vi "S7_Optimize_DB_Read_Array.vi"(2 "S7 Read Array Input":T3[](array[typedef]) {"Address Areas" items=["I/O (P)"=128, "Input (I)"=129, "Output (Q)"=130, "Bit Memory (M)"=131, "Data (DB)"=132, "Instance Data (DI)"=133, "Local Data (L)"=134, "Predecessor Local Data (VL)"=135]; "Read / Write" items=["Read"=4, "Write"=5]; "Bit Number / Byte Length" max=7 step=1}, 3 "Max Size":u8=222) -> (0 "Optimized Data Index":T1[](array[typedef]) {"Bit Number" max=7 step=1}, 1 "Optimized S7 Read Array Output":T3[](array[typedef]) {"Address Areas" items=["I/O (P)"=128, "Input (I)"=129, "Output (Q)"=130, "Bit Memory (M)"=131, "Data (DB)"=132, "Instance Data (DI)"=133, "Local Data (L)"=134, "Predecessor Local Data (VL)"=135]; "Read / Write" items=["Read"=4, "Write"=5]; "Bit Number / Byte Length" max=7 step=1})   [LabVIEW 2014, in "S7 TCP.lvlib"]
uses:
  S7 TCP.lvlib
  Data Type.ctl
  S7 Read Write Cluster.ctl
  Optimized Data Index.ctl
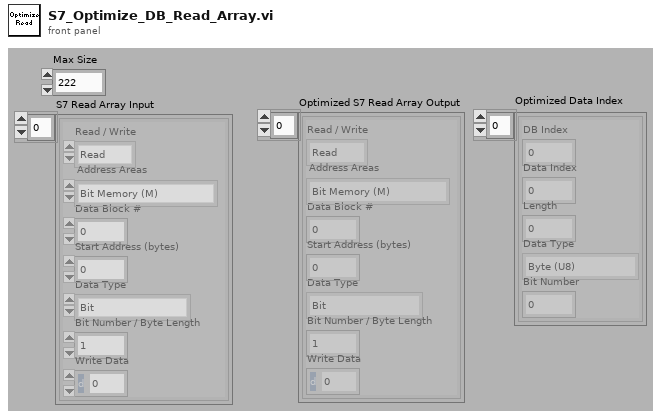
[diagram p1: front panel]
types:
  T1 = typedef "S7 TCP.lvlib/Optimized Data Index.ctl" = cluster{"DB Index":i32, "Data Index":i32, "Length":i32, "Data Type":T2, "Bit Number":u8}
  T2 = typedef "S7 TCP.lvlib/Data Type.ctl" = enum16{"Bit", "Byte (U8)", "Signed Byte (I8)", "Word (U16)", "Signed Word (I16)", "Long (U32)", "Signed Long (I32)", "Real (SGL)", "Defined Byte Length"}
  T3 = typedef "S7 TCP.lvlib/S7 Read Write Cluster.ctl" = cluster{"Read / Write":u8, "Address Areas":u8, "Data Block #":u16, "Start Address (bytes)":u32, "Data Type":T2, "Bit Number / Byte Length":u8, "Write Data":dbl}
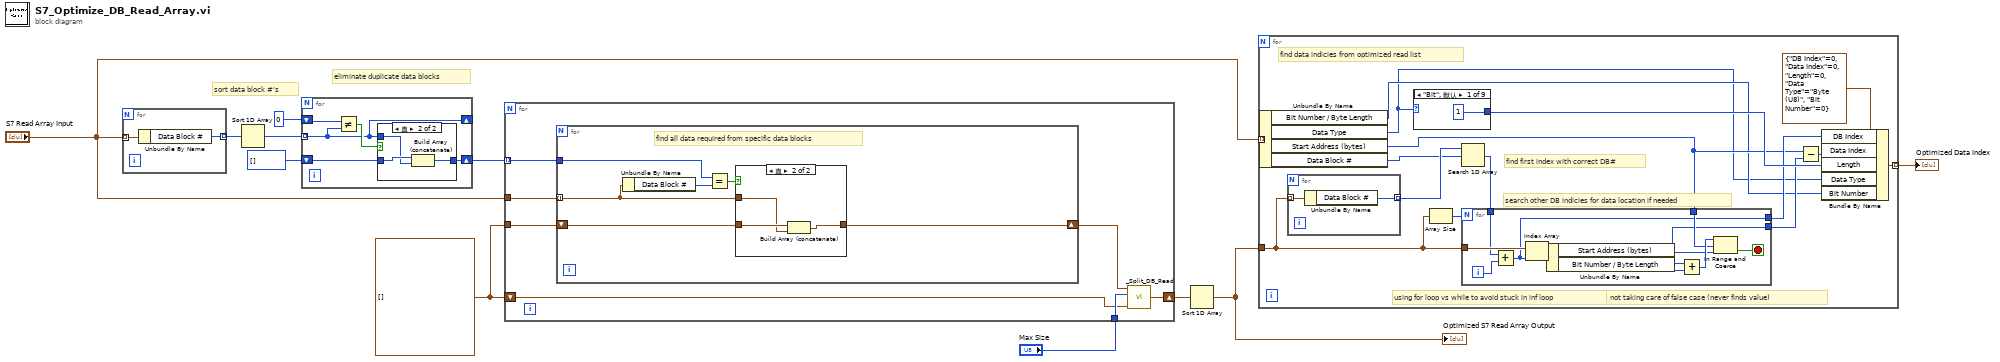
[diagram p0: block diagram]
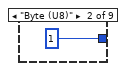
[diagram p2: hidden frame]
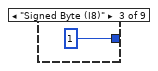
[diagram p3: hidden frame]
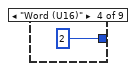
[diagram p4: hidden frame]
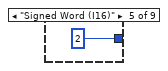
[diagram p5: hidden frame]
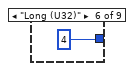
[diagram p6: hidden frame]
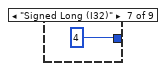
[diagram p7: hidden frame]
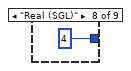
[diagram p8: hidden frame]
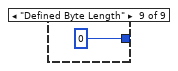
[diagram p9: hidden frame]
diagram:
  w2 = T3[] [] ("Optimized S7 Read Array Output 2")
  # "eliminate duplicate data blocks"
  # "sort data block #'s"
  n1 = for {
    tunnel: "S7 Read Array Input" -> [w13] mode=indexing
    tunnel: [w12] -> w11 mode=indexing
    n2 = Unbundle By Name(w13) -> ("Data Block #"=w12:u16)
  }
  n3 = Sort 1D Array(array=w11) -> (sorted array=w10:u16[])
  n4 = for {
    tunnel: w10 -> [w14] mode=indexing
    shift-right: [w16] -> w7
    shift-left: u16[] [] -> [w15]
    shift-right: [w14] -> _
    shift-left: u16 0 -> [w18]
    n5 = Not Equal?(x=w18, y=w14) -> (x != y?=w17:bool)
    n6 = case shown="真" w17 {
      tunnel: [w19 w22] -> w16
      tunnel: w15 -> [w19 w21]
      tunnel: w14 -> [_ w20]
      frame False {
      }
      frame True {
        n7 = Build Array (concatenate)(w21, w20) -> (w22:u16[])
      }
    }
  }
  n8 = for {
    tunnel: w7 -> [w28] mode=indexing
    tunnel: "S7 Read Array Input" -> [w29]
    tunnel: w2 -> [w27]
    tunnel: "Max Size" -> [w25]
    shift-right: [w24] -> w3
    shift-left: w2 -> [w23]
    n9 = for {
      tunnel: w29 -> [w35] mode=indexing
      tunnel: w28 -> [w31]
      shift-right: [w32] -> w26
      shift-left: w27 -> [w33]
      # "find all data required from specific data blocks"
      n10 = Unbundle By Name(w35) -> ("Data Block #"=w30:u16)
      n11 = Equal?(x=w31, y=w30) -> (x = y?=w34:bool)
      n12 = case shown="真" w34 {
        tunnel: w35 -> [_ w37]
        tunnel: w33 -> [w36 w39]
        tunnel: [w36 w38] -> w32
        frame False {
        }
        frame True {
          n13 = Build Array (concatenate)(w39, w37) -> (w38:T3[])
        }
      }
    }
    n14 = call "_Split_DB_Read.vi"("Lists of S7 Read Items"=w26, "Max Size"=w25, "S7 Read Array Input"=w23) -> ("Optimized S7 Read Array Output"=w24:T3[])  [unwired: 1 in, 1 out]
  }
  n15 = Sort 1D Array(array=w3) -> (sorted array=w1:T3[])
  "Optimized S7 Read Array Output" <- w1
  n16 = for {
    tunnel: w1 -> [w47]
    tunnel: "S7 Read Array Input" -> [w54] mode=indexing
    tunnel: [w45] -> w5 mode=indexing
    # "find data indicies from optimized read list"
    # "search other DB indicies for data location if needed"
    # "find first index with correct DB#"
    # "using for loop vs while to avoid stuck in inf loop"
    # "warning - not taking care of false case (never finds value)"
    n17 = Unbundle By Name(w54) -> ("Bit Number / Byte Length"=w41:u8, "Data Type"=w40:T2, "Start Address (bytes)"=w44:u32, "Data Block #"=w52:u16)
    n18 = for {
      tunnel: w47 -> [w75] mode=indexing
      tunnel: [w74] -> w53 mode=indexing
      n19 = Unbundle By Name(w75) -> ("Data Block #"=w74:u16)
    }
    n20 = case shown="\"Bit\", 默认" w40 {
      tunnel: [u8 1 ("Bit Number / Byte Length") u8 1 ("Bit Number / Byte Length") u8 1 ("Bit Number / Byte Length") u8 2 ("Bit Number / Byte Length") u8 2 ("Bit Number / Byte Length") u8 4 ("Bit Number / Byte Length") u8 4 ("Bit Number / Byte Length") u8 4 ("Bit Number / Byte Length") u8 0 ("Bit Number / Byte Length")] -> w49
      frame "Bit", Default {
      }
      frame "Byte (U8)" {
      }
      frame "Signed Byte (I8)" {
      }
      frame "Word (U16)" {
      }
      frame "Signed Word (I16)" {
      }
      frame "Long (U32)" {
      }
      frame "Signed Long (I32)" {
      }
      frame "Real (SGL)" {
      }
      frame "Defined Byte Length" {
      }
    }
    n21 = Array Size(array=w47) -> (size(s)=w48:i32)
    n22 = Search 1D Array(1D array=w53, element=w52) -> (index of element=w51:i32)  [unwired: 1 out]
    n23 = for {
      N: w48 -> [_]
      tunnel: w47 -> [w64]
      tunnel: w51 -> [w63]
      tunnel: w44 -> [w59]
      tunnel: [w56] -> w46
      tunnel: [w55] -> w43
      i -> [w57]
      stop <- w58 stop-if-true
      n24 = Add(x=w63, y=w57) -> (x+y=w56:i32)
      n25 = Index Array(array=w64, index=w56) -> (element=w62:T3)
      n26 = Unbundle By Name(w62) -> ("Start Address (bytes)"=w55:u32, "Bit Number / Byte Length"=w61:u8)
      n27 = Add(x=w61, y=w55) -> (x+y=w60:u32)
      n28 = In Range and Coerce(upper limit=w60, x=w59, lower limit=w55) -> (In Range?=w58:bool)  [unwired: 1 out]
    }
    n29 = Subtract(x=w44, y=w43) -> (x-y=w42:u32)
    n30 = Bundle By Name(cluster=T1 {"DB Index"=0, "Data Index"=0, "Length"=0, "Data Type"=enum."Byte (U8)", "Bit Number"=0} ("Cluster"), "DB Index"=w46, "Data Index"=w42, "Length"=w49, "Data Type"=w40, "Bit Number"=w41) -> (w45:T1)
  }
  "Optimized Data Index" <- w5
